vi "Generate SQL Values.vi"(8 "error in (no error)":errorcluster, 11 "Transaction in":refnum<class "Transaction.lvclass">) -> (0 "error out":errorcluster, 2 "SQL Values":string, 3 "Transaction out":refnum<class "Transaction.lvclass">)   [LabVIEW 2018, in "Transaction.lvclass"]
uses:
  Transaction.lvclass
  Transaction.lvclass/Transaction.ctl
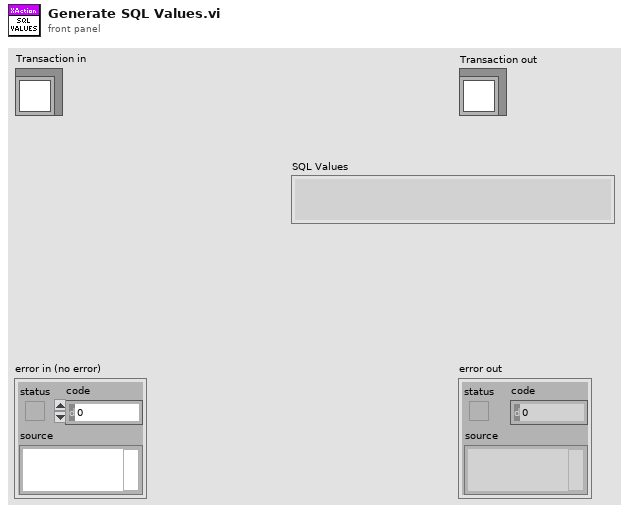
[diagram p1: front panel]
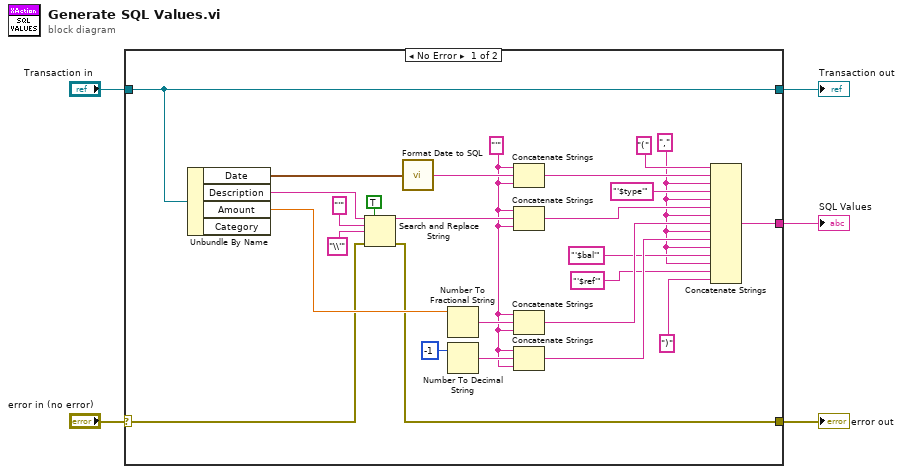
[diagram p0: block diagram]
diagram:
  n1 = case shown="No Error" "error in (no error)" {
    selector: "error in (no error)" -> [w20 w33]
    tunnel: [w19 w33] -> w4
    tunnel: "Transaction in" -> [w18 w32]
    tunnel: [w18 w32] -> w2
    tunnel: [w17 _] -> w1
    frame No Error {
      w9 = "'"
      w6 = ","
      n2 = Unbundle By Name(w18) -> ("Date"=w16:timestamp, "Description"=w23:string, "Amount"=w22:dbl)  [unwired: 1 out]
      n3 = Search and Replace String(replace all?=TRUE ("replace all? (F)"), input string=w23, search string="'", replace string="\\'", error in=w20) -> (result string=w25:string, error out=w19:errorcluster)  [unwired: 5 out]
      n4 = call "Format Date to SQL.vi"("Date"=w16) -> ("SQL Date"=w15:string)
      n5 = Number To Fractional String(number=w22) -> (F-format string=w21:string)  [unwired: 3 in]
      n6 = Number To Decimal String(number=-1) -> (decimal integer string=w12:string)  [unwired: 1 in]
      n7 = Concatenate Strings(w9, w15, w9) -> (w26:string)
      n8 = Concatenate Strings(w9, w25, w9) -> (w27:string)
      n9 = Concatenate Strings(w9, w21, w9) -> (w28:string)
      n10 = Concatenate Strings(w9, w12, w9) -> (w13:string)
      n11 = Concatenate Strings("(", w26, w6, "'$type'", w6, w27, w6, w28, w6, w13, w6, "'$bal'", w6, "'$ref'", ")") -> (w17:string)
    }
    frame Error {
    }
  }
  "error out" <- w4
  "Transaction out" <- w2
  "SQL Values" <- w1
